vi "ZY to Y1.vi"(10 "ZY_control":T3 {"Y_H" step=1.0; "SP" step=0.01 format="%.2f"}) -> (2 "Y":T1={"Y_HSw"=1, "Y_HSetState"=enum."initialize", "Y_ASetState"=enum."initialize", "Y_DSetState"=enum."initialize"})   [LabVIEW 2019, in "Heating.lvlib"]
uses:
  ctl/ZY_control.ctl
  ctl/Z_State.ctl
  ctl/Y_state.ctl
  ctl/Y_control.ctl
  Heating.lvlib
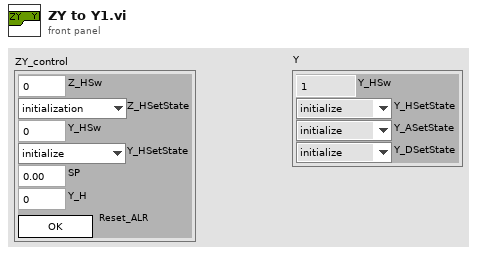
[diagram p1: front panel]
types:
  T1 = typedef "Heating.lvlib/Y_control.ctl" = cluster{"Y_HSw":u8, "Y_HSetState":T2, "Y_ASetState":T2, "Y_DSetState":T2}
  T2 = typedef "Heating.lvlib/Y_state.ctl" = enum8{"initialize", "alarm", "min", "stop", "hand", "auto", "max"}
  T3 = typedef "Heating.lvlib/ZY_control.ctl" = cluster{"Z_HSw":u8, "Z_HSetState":T4, "Y_HSw":u8, "Y_HSetState":T2, "SP":dbl, "Y_H":dbl, "Reset_ALR":bool}
  T4 = typedef "Heating.lvlib/Z_State.ctl" = enum8{"initialization", "alarm", "disabled", "not ready", "stop ready", "reserv", "switched off", "reserv2", "switched on", "check", "on min", "decrease out", "on", "increase out", "on max"}
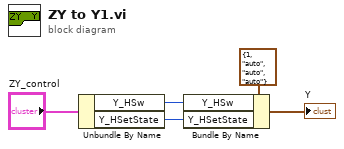
[diagram p0: block diagram]
diagram:
  n1 = Unbundle By Name("ZY_control") -> ("Y_HSw"=w3:u8, "Y_HSetState"=w2:T2)
  n2 = Bundle By Name(cluster=T1 {"Y_HSw"=1, "Y_HSetState"=enum."auto", "Y_ASetState"=enum."auto", "Y_DSetState"=enum."auto"} ("Y"), "Y_HSw"=w3, "Y_HSetState"=w2) -> (→"Y":T1)
